vi "CC Focus GUI.vi"(9 "Standalone":bool=TRUE, 10 "Init Data":variant, 11 "Name":string) -> ()   [LabVIEW 2024]
uses:
  typedefs/CC enum Operation Mode.ctl
  Focus cluster Settings.ctl
  Focus Hardware Types.ctl
  Focus cluster Motion Settings.ctl
  Focus Class/Focus Class.lvclass
  Subsystems/SS typedef cluster Instrument Command Queue Data.ctl
  Subsystems/SS cluster Data Queue type.ctl
  Focus cluster MoveFocus Command Parameters.ctl
  hk-channel-class/hk-channel-class/HK Item/HK Item.lvclass
  FocusSimulator/FocusSimulator.lvclass
  NewFocus/NewFocus.lvclass
  ArduinoFocus/ArduinoFocus.lvclass
  hk-channel-class/hk-channel-class/HK Item/HK Item.lvclass/HK Item.ctl
  hk-channel-class/hk-channel-class/HK Item/HK Channel cluster Telemetry Data.ctl
  hk-channel-class/hk-channel-class/HK Item/HK Channel enum Data Type.ctl
  typedefs/CC cluster Script.ctl
  typedefs/CC Script Step.ctl
  typedefs/CC enum Script Action.ctl
  Scripts/CC Rd Wr Script Action.ctl
  hk-channel-class/hk-channel-class/HK Item/Write Source.vi
  hk-channel-class/hk-channel-class/HK Item/HK Channel Read Name.vi
panel:
  out "Messages":string
  in  "Mode":T1
  in  "Tab Control":enum32{"Focus Motor", "Engineering"}(tab)
  in  "Exp Time":dbl format="%.1g"
  in  "Peform Focus Scan":bool
  in  "Images":i32=10
  in  "Motor 1 Steps":i32
  in  "Motor 0 Steps":i32
  in  "Absolute":bool
  in  "Relative":bool
  in  "Steps":i32
  out "Controller Name":string
  in  "Select Motor (0:n-1)":i32 min=0 max=3 step=1
  out "Positions":i32[](array[slide]) scale=-10000.0..10000.0
  in  "Error":bool
  out "Homed":bool[](array[boolean])
  in  "STOP":bool
  out "Connected":bool
  in  "Close":bool
  in  "Home":bool
  in  "Configure":bool
  in  "Reset Startup Positions":bool
  in  "Connect":bool
  in  "Focus Settings":T2
  in  "Power Up Positions":i32[](array[numeric])
  # "Click for info"
  # "We need to remember where we were last in case\npower cycled on NewFocus controller. Change\ncode to use saved positions only if controller reports\nall 0s for position."
  # "Factory Settings: \nVelocity 1750 Steps/sec\nAcceleration 100000 Steps/sec/sec"
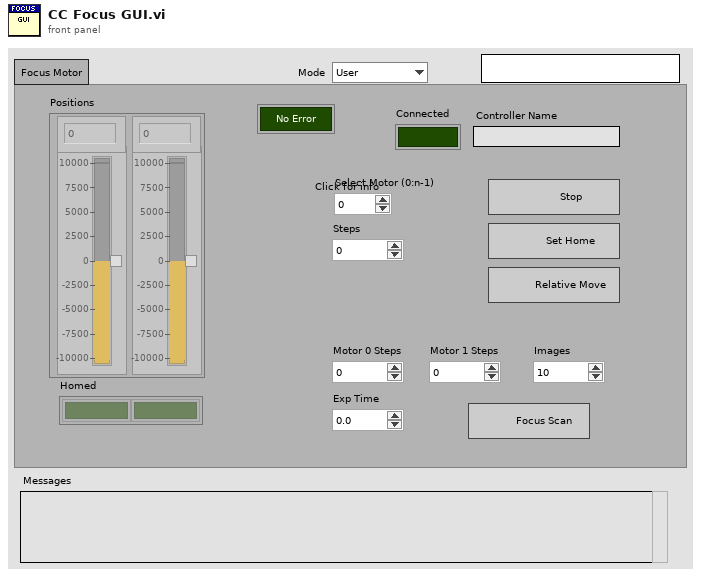
[diagram p1: front panel]
types:
  T1 = typedef "CC enum Operation Mode.ctl" = enum16{"User", "Engineering"}
  T2 = typedef "Focus cluster Settings.ctl" = cluster{"Type":T3, "Motion Settings":T4, "Last Positions":i32[]}
  T3 = typedef "Focus Hardware Types.ctl" = enum16{"Simulated", "NewFocus", "Arduino"}
  T4 = typedef "Focus cluster Motion Settings.ctl" = cluster{"Steps Per Sec":i32, "Steps Per Sec 2":i32}
  T5 = typedef "SS typedef cluster Instrument Command Queue Data.ctl" = cluster{"Cmd":string, "Parameters":variant}
  T6 = typedef "Focus cluster MoveFocus Command Parameters.ctl" = cluster{"Motor":i32, "Position":i32}
  T7 = cluster{"state":refnum<user-event>, "Focus Settings":T2, "Focus Ref":refnum<class "Focus Class.lvclass">, "Error":errorcluster, "Msg":string, "Start Pos":i32[], "cmd q":refnum<queue>, "data q":refnum<queue>, "next poll":timestamp, "Cmd":T5, "move":T6, "Name":string, "send time":timestamp, "Focus Script":string, "Ch List":refnum<class "HK Item.lvclass">[], "move names":string[], "pos names":string[], "Prev data":i32[]}
  T8 = typedef "SS cluster Data Queue type.ctl" = cluster{"Source":string, "Type":string, "Data":variant}
  T9 = typedef "HK Item.lvclass/HK Channel enum Data Type.ctl" = enum16{"Floating Point", "Integer", "Enum", "String", "Waveform", "File"}
  T10 = typedef "HK Item.lvclass/HK Channel cluster Telemetry Data.ctl" = cluster{"Ch Names":string[], "Ch Values":dbl[], "Timestamp":timestamp, "Data Type":T9}
  T11 = typedef "CC Rd Wr Script Action.ctl" = enum16{"Read", "Write", "List", "Delete"}
  T12 = typedef "CC cluster Script.ctl" = cluster{"Name":string, "Script":T13[]}
  T13 = typedef "CC Script Step.ctl" = cluster{"Action":T14, "Data":variant}
  T14 = typedef "CC enum Script Action.ctl" = enum16{"Noop", "Define Object", "Define Exposure", "Define Dithering", "Acquire Images", "Set Filter Wheel", "Telescope Home", "Telescope Move", "Telescope RA DEC", "Focus Move Relative", "Focus Move Absolute", "Focus Set Home", "Macro", "Pause", "Ask User", "Define Random Dither", "CmdLine", "Outlet"}
  T15 = typedef "CC cluster Script Panel Defaults.ctl" = cluster{"Script Name":string, "Script Path":path}
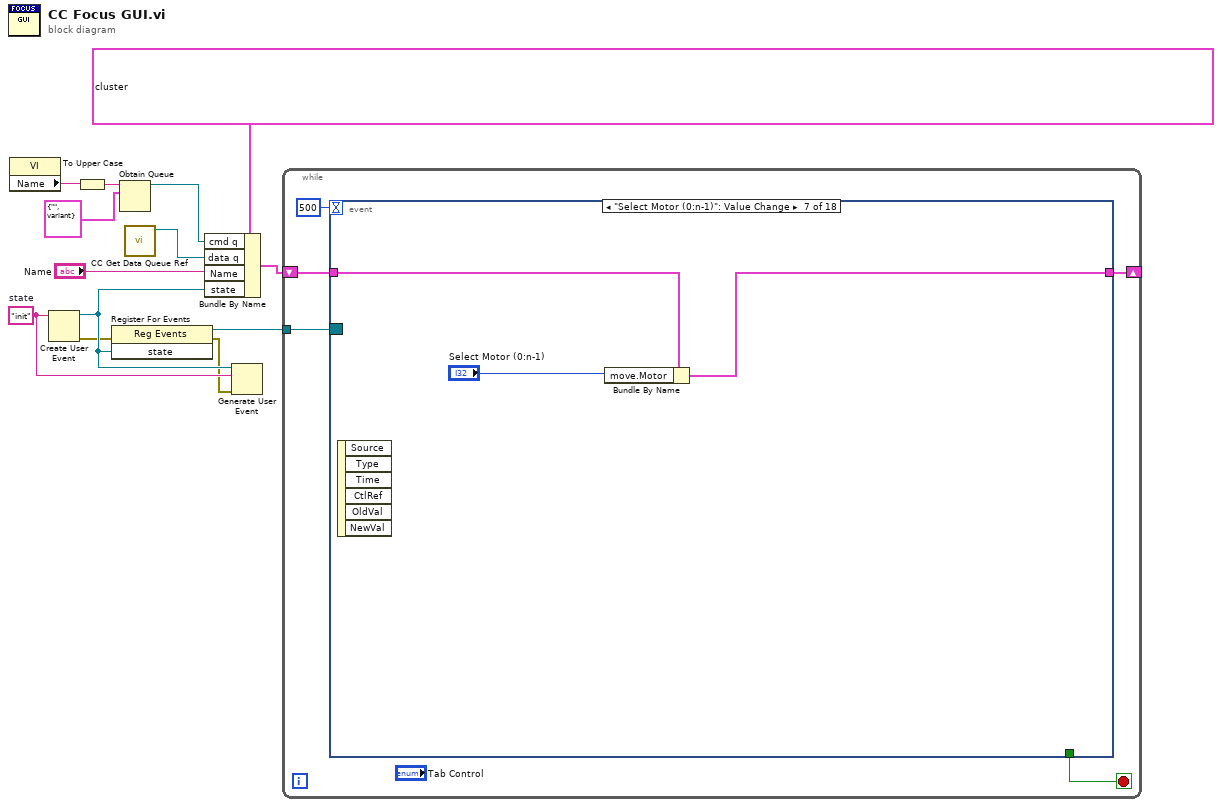
[diagram p0: block diagram]
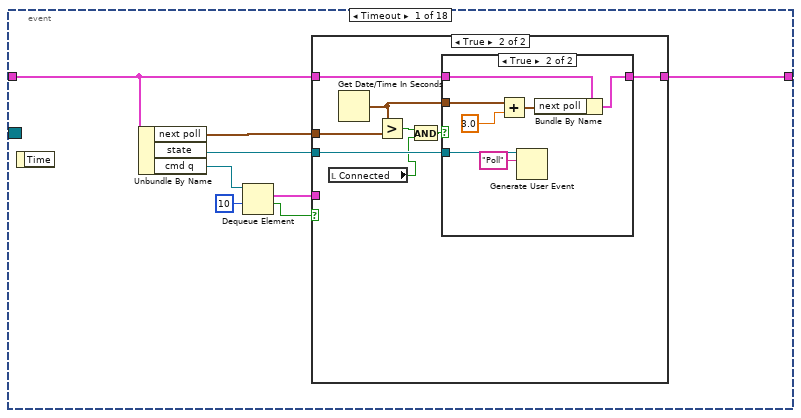
[diagram p2: hidden frame]
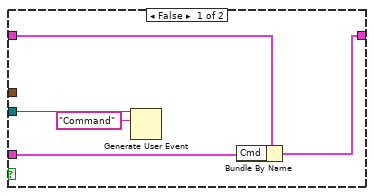
[diagram p3: hidden frame]
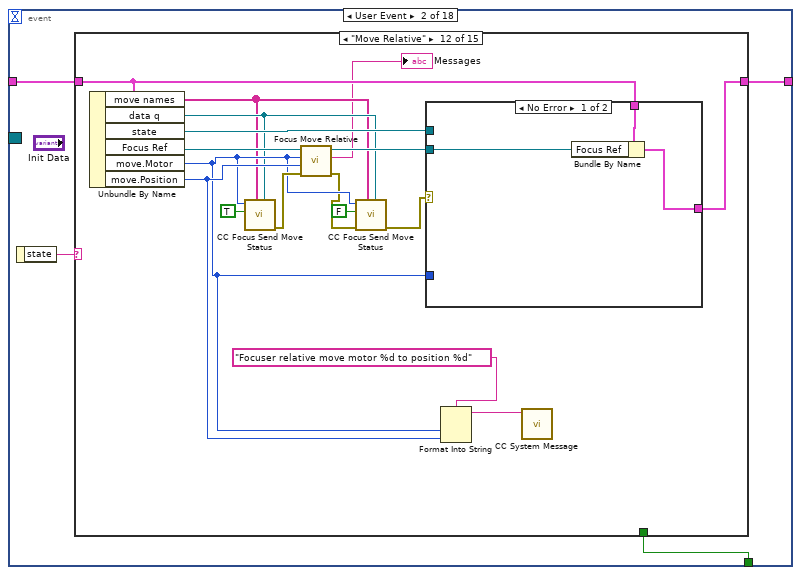
[diagram p5: hidden frame]
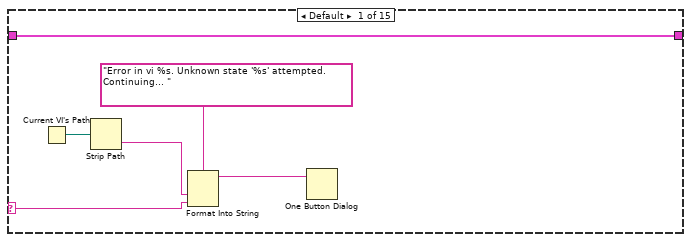
[diagram p6: hidden frame]
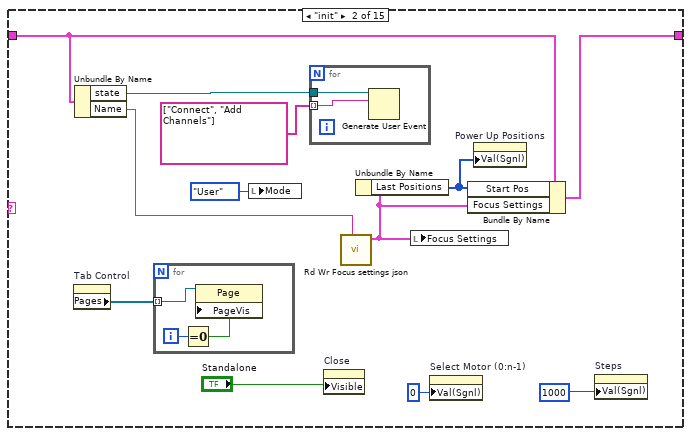
[diagram p7: hidden frame]
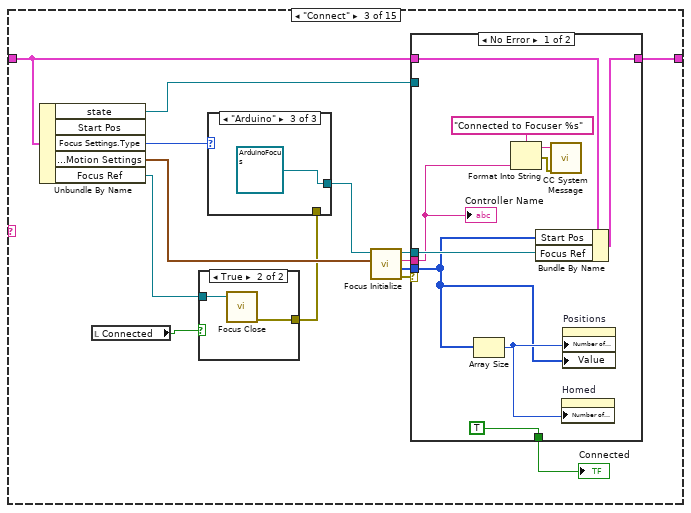
[diagram p8: hidden frame]
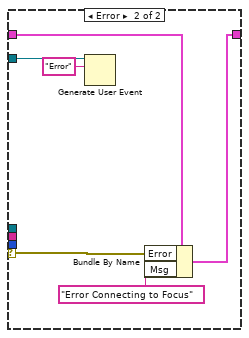
[diagram p10: hidden frame]
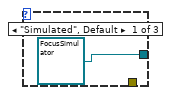
[diagram p11: hidden frame]
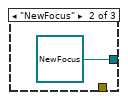
[diagram p12: hidden frame]
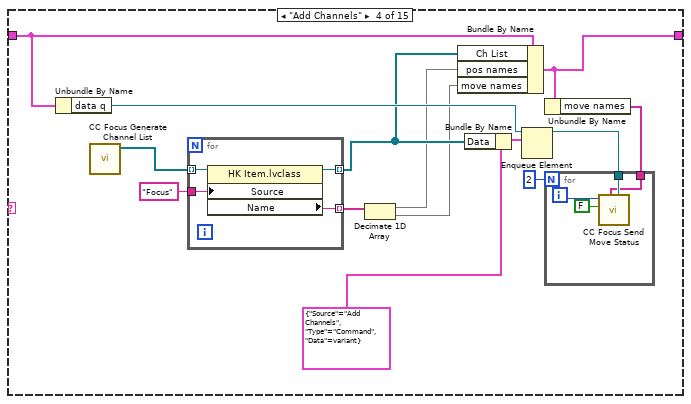
[diagram p13: hidden frame]
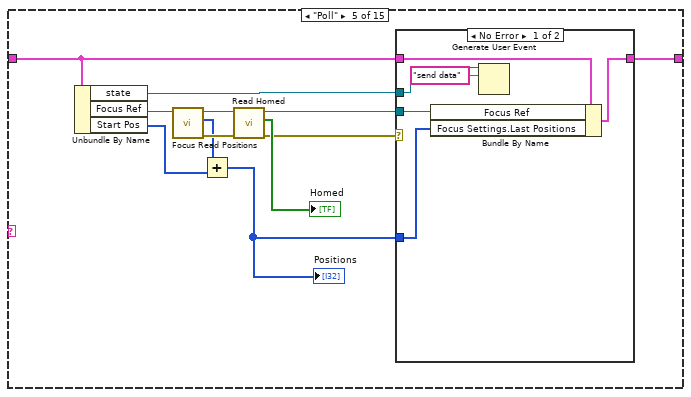
[diagram p14: hidden frame]
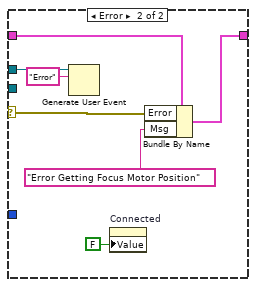
[diagram p15: hidden frame]
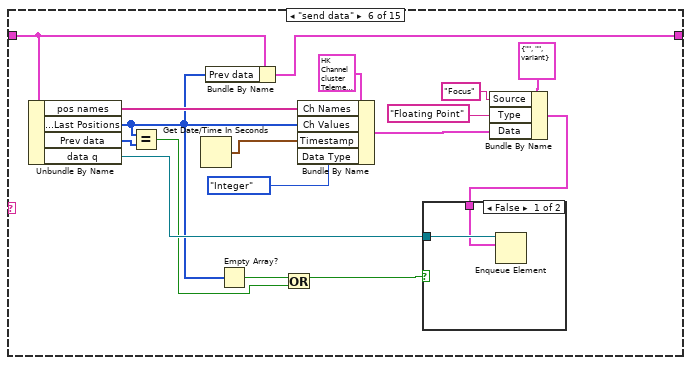
[diagram p16: hidden frame]
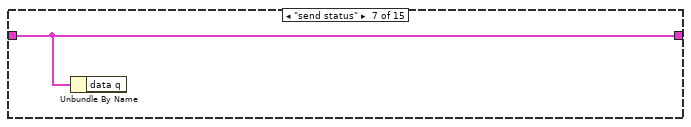
[diagram p18: hidden frame]
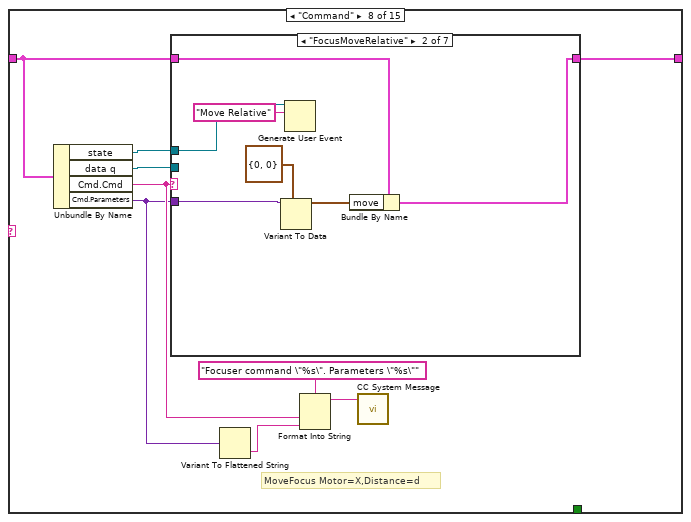
[diagram p19: hidden frame]
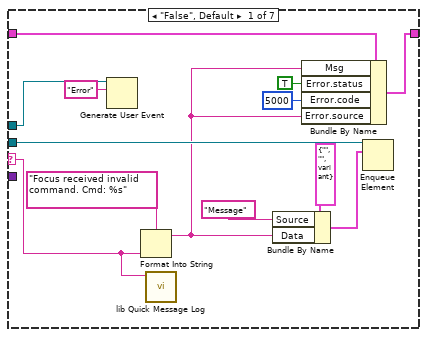
[diagram p20: hidden frame]
diagram:
  w9 = "init"  # state
  n1 = property class="VI"() -> ("Name"=w6:string)  [unwired: 2 in, 2 out]
  n2 = Create User Event(user event datatype=w9) -> (user event=w11:refnum<user-event>, error out=w7:errorcluster)  [unwired: 1 in]
  n3 = To Upper Case(1:w6) -> (0:w5:string)
  n4 = register-events(error in=w7, w11) -> (reference out=w10:refnum<event-registration>, error out=w8:errorcluster)  [unwired: 1 in]
  n5 = Obtain Queue(name (unnamed)=w5, element data type=T5 {"Cmd"="", "Parameters"=variant}) -> (queue out=w3:refnum<queue>)  [unwired: 3 in, 2 out]
  n6 = call "CC Get Data Queue Ref.vi"() -> ("Data Q"=w2:refnum<queue>)  [unwired: 10 in, 1 out]
  n7 = Bundle By Name(cluster=T7 {"state"=refnum, "Focus Settings"={"Type"=enum."Simulated", "Motion Settings"={"Steps Per Sec"=0, "Steps Per Sec 2"=0}, "Last Positions"=[]}, "Focus Ref"=refnum, "Error"={"status"=FALSE, "code"=0, "source"=""}, "Msg"="", "Start Pos"=[], "cmd q"=refnum, "data q"=refnum, "next poll"=timestamp(0 s since 1904-01-01), "Cmd"={"Cmd"="", "Parameters"=variant}, "move"={"Motor"=0, "Position"=0}, "Name"="NewFocus", "send time"=timestamp(0 s since 1904-01-01), "Focus Script"="", "Ch List"=[], "move names"=[], "pos names"=[], "Prev data"=[]}, "cmd q"=w3, "data q"=w2, "Name"="Name", "state"=w11) -> (w12:T7)
  n8 = Generate User Event(user event=w11, event data cluster=w9, error in=w8) -> ()  [unwired: 1 in, 2 out]
  n9 = while {
    tunnel: w10 -> [w18]
    shift-right: [w16] -> _
    shift-left: w12 -> [w17]
    stop <- w15 stop-if-true
    n10 = event shown="[6] \"Select Motor (0:n-1)\": Value Change" {
      selector: w18 -> [_ _ _ _ _ _ _ _ _ _ _ _ _ _ _ _ _ _]
      dyn-events: _ -> [_ _ _ _ _ _ _ _ _ _ _ _ _ _ _ _ _ _]
      timeout: 500 -> [_ _ _ _ _ _ _ _ _ _ _ _ _ _ _ _ _ _]
      tunnel: w17 -> [w20 w50 w338 w356 w362 w374 w378 w381 w387 w390 w393 w396 w397 w407 w417 w420 w434 w437]
      tunnel: [w19 w49 w340 w357 w362 w375 w379 w382 w387 w390 w393 w396 w398 w408 w417 w421 w434 w437] -> w16
      tunnel: [_ w48 _ _ _ _ _ _ _ _ _ _ _ _ _ _ _ _] -> w15
      event Timeout {
        n11 = event-data() -> ()  [unwired: 1 in, 1 out]
        n12 = Unbundle By Name(w20) -> ("next poll"=w21:timestamp, "state"=w22:refnum<user-event>, "cmd q"=w26:refnum<queue>)
        n13 = Dequeue Element(queue=w26, timeout in ms (-1)=10) -> (element=w23:T5, timed out?=w24:bool)  [unwired: 1 in, 2 out]
        n14 = case shown="True" w24 {
          tunnel: w23 -> [w28 _]
          tunnel: w22 -> [w31 w36]
          tunnel: w20 -> [w29 w37]
          tunnel: [w27 w34] -> w19
          tunnel: w21 -> [_ w39]
          frame False {
            n15 = Generate User Event(user event=w31, event data cluster="Command" ("event data")) -> ()  [unwired: 2 in, 2 out]
            n16 = Bundle By Name(cluster=w29, "Cmd"=w28) -> (w27:T7)
          }
          frame True {
            n17 = local read "Connected"() -> (w32:bool)
            n18 = Get Date/Time In Seconds() -> (seconds since 1Jan1904=w35:timestamp)
            n19 = Greater?(x=w35, y=w39) -> (0:w38:bool)
            n20 = And(x=w38, y=w32) -> (x .and. y?=w33:bool)
            n21 = case shown="True" w33 {
              tunnel: w37 -> [w40 w47]
              tunnel: w36 -> [_ w46]
              tunnel: w35 -> [_ w45]
              tunnel: [w40 w42] -> w34
              frame False {
              }
              frame True {
                n22 = Add(x=w45, y=3.0) -> (x+y=w43:timestamp)
                n23 = Generate User Event(user event=w46, event data cluster="Poll" ("event data")) -> ()  [unwired: 2 in, 2 out]
                n24 = Bundle By Name(cluster=w47, "next poll"=w43) -> (w42:T7)
              }
            }
          }
        }
      }
      event User Event {
        n25 = event-data() -> ("state"=w51:string)  [unwired: 1 in]
        n26 = case shown="\"Move Relative\"" w51 {
          selector: w51 -> [w56 _ _ _ _ _ _ _ _ _ _ _ _ _ _]
          tunnel: w50 -> [w52 w66 w84 w118 w137 w157 w176 w182 w234 w241 w259 w287 w307 w328 w335]
          tunnel: [w52 w67 w85 w112 w136 w158 w176 w183 w234 w242 w260 w288 w308 w328 w335] -> w49
          tunnel: [_ _ _ _ _ _ _ _ _ _ _ _ _ TRUE _] -> w48
          frame Default {
            n27 = Current VI's Path() -> (path=w55:path)
            n28 = Strip Path(path=w55) -> (name=w54:string)  [unwired: 1 out]
            n29 = Format Into String(format string="Error in vi %s. Unknown state '%s' attempted. Continuing... ", w54, w56) -> (resulting string=w53:string)  [unwired: 2 in, 1 out]
            n30 = One Button Dialog(message=w53) -> ()  [unwired: 1 in, 1 out]
          }
          frame "init" {
            n31 = property on="Tab Control" class="TabCtl (strict)"() -> ("Pages"=w58:refnum<vi>[])  [unwired: 2 in, 2 out]
            n32 = Unbundle By Name(w66) -> ("state"=w69:refnum<user-event>, "Name"=w60:string)
            n33 = for {
              tunnel: w58 -> [w72] mode=indexing
              i -> [w71]
              n34 = Equal To 0?(x=w71) -> (x = 0?=w70:bool)
              n35 = property class="Page"(reference=w72, "PageVis"=w70) -> ()  [unwired: 1 in, 2 out]
            }
            n36 = local write "Mode"(CC_enum_Operation_Mode."User" ("Mode")) -> ()
            n37 = for {
              tunnel: w69 -> [w74]
              tunnel: string[] ["Connect", "Add Channels"] -> [w73] mode=indexing
              n38 = Generate User Event(user event=w74, event data cluster=w73) -> ()  [unwired: 2 in, 2 out]
            }
            n39 = property on="Close" class="Bool"("Visible"="Standalone") -> ()  [unwired: 2 in, 2 out]
            n40 = call "Rd Wr Focus settings json.vi"("Focus Name"=w60) -> ("Focus Settings"=w62:T2)  [unwired: 9 in, 1 out]
            n41 = Unbundle By Name(w62) -> ("Last Positions"=w61:i32[])
            n42 = local write "Focus Settings"(w62) -> ()
            n43 = property on="Select Motor (0:n-1)" class="DigNum (strict)"("Val(Sgnl)"=0 ("Value (Signaling)")) -> ()  [unwired: 2 in, 2 out]
            n44 = Bundle By Name(cluster=w66, "Start Pos"=w61, "Focus Settings"=w62) -> (w67:T7)
            n45 = property on="Power Up Positions" class="Arr (strict)"("Val(Sgnl)"=w61) -> ()  [unwired: 2 in, 2 out]
            n46 = property on="Steps" class="DigNum (strict)"("Val(Sgnl)"=1000 ("Steps")) -> ()  [unwired: 2 in, 2 out]
          }
          frame "Connect" {
            n47 = Unbundle By Name(w84) -> ("state"=w81:refnum<user-event>, "Focus Settings.Type"=w88:T3, "Focus Settings.Motion Settings"=w83:T4, "Focus Ref"=w77:refnum<class "Focus Class.lvclass">)  [unwired: 1 out]
            n48 = local read "Connected"() -> (w78:bool)
            n49 = case shown="True" w78 {
              tunnel: w77 -> [_ w90]
              tunnel: [_ w89] -> w76
              frame False {
              }
              frame True {
                n50 = call-dynamic "Focus Close.vi"("Focus Class in"=w90) -> ("error out"=w89:errorcluster)  [unwired: 9 in, 1 out]
              }
            }
            n51 = case shown="\"Arduino\"" w88 {
              tunnel: [refnum<class "FocusSimulator.lvclass"> refnum ("FocusSimulator.lvclass") refnum<class "NewFocus.lvclass"> refnum ("NewFocus.lvclass") refnum<class "ArduinoFocus.lvclass"> refnum ("ArduinoFocus.lvclass")] -> w87
              tunnel: w76 -> [_ _ _]
              frame "Simulated", Default {
              }
              frame "NewFocus" {
              }
              frame "Arduino" {
              }
            }
            n52 = call-dynamic "Focus Initialize.vi"("Motion Settings"=w83, "Focus Class in"=w87) -> ("error out"=w82:errorcluster, "Motor Positions"=w75:i32[], "Device Name"=w80:string, "Focus Class out"=w86:refnum<class "Focus Class.lvclass">)  [unwired: 6 in]
            n53 = case shown="No Error" w82 {
              selector: w82 -> [_ w105]
              tunnel: w86 -> [w100 _]
              tunnel: [w99 w104] -> w85
              tunnel: w84 -> [w98 w106]
              tunnel: w81 -> [_ w103]
              tunnel: w80 -> [w93 _]
              tunnel: [TRUE _] -> w79
              tunnel: w75 -> [w91 _]
              frame No Error {
                n54 = Array Size(array=w91) -> (size(s)=w92:i32)
                n55 = Format Into String(format string="Connected to Focuser %s", w93) -> (resulting string=w94:string, error out=w96:errorcluster)  [unwired: 2 in]
                n56 = Bundle By Name(cluster=w98, "Start Pos"=w91, "Focus Ref"=w100) -> (w99:T7)
                n57 = call "CC System Message.vi"("error in (no error)"=w96, "Message"=w94) -> ()  [unwired: 9 in, 1 out]
                n58 = property on="Homed" class="Arr (strict)"("Number of Columns"=w92) -> ()  [unwired: 2 in, 2 out]
                n59 = property on="Positions" class="Arr (strict)"("Number of Columns"=w92, "Value"=w91) -> ()  [unwired: 2 in, 2 out]
                "Controller Name" <- w93
              }
              frame Error {
                n60 = Generate User Event(user event=w103, event data cluster="Error" ("event data")) -> ()  [unwired: 2 in, 2 out]
                n61 = Bundle By Name(cluster=w106, "Error"=w105, "Msg"="Error Connecting to Focus") -> (w104:T7)
              }
            }
            "Connected" <- w79
          }
          frame "Add Channels" {
            n62 = Unbundle By Name(w118) -> ("data q"=w121:refnum<queue>)
            n63 = call "CC Focus Generate Channel List.vi"() -> ("Channel List"=w117:refnum<class "HK Item.lvclass">[])  [unwired: 9 in, 2 out]
            n64 = for {
              tunnel: w117 -> [w131] mode=indexing
              tunnel: [w130] -> w120 mode=indexing
              tunnel: "Focus" ("Name") -> [w129]
              tunnel: [w128] -> w116 mode=indexing
              n65 = property class="HK Item.lvclass"(reference=w131, "Source"=w129) -> (reference out=w130:refnum<class "HK Item.lvclass">, "Name"=w128:string)  [unwired: 1 in, 1 out]
            }
            n66 = Decimate 1D Array(w116) -> (w115:string[], w114:string[])
            n67 = Bundle By Name(cluster=w118, "Ch List"=w120, "pos names"=w115, "move names"=w114) -> (w112:T7)
            n68 = Bundle By Name(cluster=T8 {"Source"="Add Channels", "Type"="Command", "Data"=variant} ("element"), "Data"=w120) -> (w123:T8)
            n69 = Enqueue Element(queue=w121, element=w123) -> (queue out=w113:refnum<queue>)  [unwired: 2 in, 2 out]
            n70 = Unbundle By Name(w112) -> ("move names"=w111:string[])
            n71 = for {
              N: 2 -> [_]
              tunnel: w113 -> [w126]
              tunnel: w111 -> [w124]
              i -> [w125]
              n72 = call "CC Focus Send Move Status.vi"("data q"=w126, "Names"=w124, "Moving"=FALSE, "motor"=w125) -> ()  [unwired: 7 in, 1 out]
            }
          }
          frame "Poll" {
            n73 = Unbundle By Name(w137) -> ("state"=w138:refnum<user-event>, "Focus Ref"=w143:refnum<class "Focus Class.lvclass">, "Start Pos"=w132:i32[])
            n74 = call-dynamic "Focus Read Positions.vi"("Focus Class in"=w143) -> ("error out"=w141:errorcluster, "Motor Positions"=w134:i32[], "Focus Class out"=w142:refnum<class "Focus Class.lvclass">)  [unwired: 8 in]
            n75 = Add(x=w134, y=w132) -> (x+y=w133:i32[])
            "Positions" <- w133
            n76 = call-dynamic "Read Homed.vi"("error in (no error)"=w141, "Focus Class in"=w142) -> ("error out"=w139:errorcluster, "Homed"=→"Homed":bool[], "Focus Class out"=w135:refnum<class "Focus Class.lvclass">)  [unwired: 7 in]
            n77 = case shown="No Error" w139 {
              selector: w139 -> [_ w153]
              tunnel: w138 -> [w145 w155]
              tunnel: w137 -> [w147 w156]
              tunnel: [w148 w151] -> w136
              tunnel: w135 -> [w149 _]
              tunnel: w133 -> [w146 _]
              frame No Error {
                n78 = Bundle By Name(cluster=w147, "Focus Ref"=w149, "Focus Settings.Last Positions"=w146) -> (w148:T7)
                n79 = Generate User Event(user event=w145, event data cluster="send data" ("event data")) -> ()  [unwired: 2 in, 2 out]
              }
              frame Error {
                n80 = Generate User Event(user event=w155, event data cluster="Error" ("event data")) -> ()  [unwired: 2 in, 2 out]
                n81 = property on="Connected" class="Bool (strict)"("Value"=FALSE ("Connected")) -> ()  [unwired: 2 in, 2 out]
                n82 = Bundle By Name(cluster=w156, "Error"=w153, "Msg"="Error Getting Focus Motor Position") -> (w151:T7)
              }
            }
          }
          frame "send data" {
            n83 = Unbundle By Name(w157) -> ("pos names"=w163:string[], "Focus Settings.Last Positions"=w159:i32[], "Prev data"=w162:i32[], "data q"=w170:refnum<queue>)
            n84 = Equal?(x=w159, y=w162) -> (x = y?=w160:bool)
            n85 = Get Date/Time In Seconds() -> (seconds since 1Jan1904=w172:timestamp)
            n86 = Bundle By Name(cluster=w157, "Prev data"=w159) -> (w158:T7)
            n87 = Empty Array?(array=w159) -> (empty?=w164:bool)
            n88 = Or(x=w164, y=w160) -> (x .or. y?=w161:bool)
            n89 = Bundle By Name(cluster=T10 {"Ch Names"=[], "Ch Values"=[], "Timestamp"=timestamp(0 s since 1904-01-01), "Data Type"=enum."Floating Point"}, "Ch Names"=w163, "Ch Values"=w159, "Timestamp"=w172, "Data Type"=HK_Channel_enum_Data_Type."Integer") -> (w166:T10)
            n90 = Bundle By Name(cluster=T8 {"Source"="", "Type"="", "Data"=variant} ("element"), "Source"="Focus", "Type"="Floating Point" ("Data Type"), "Data"=w166) -> (w165:T8)
            n91 = case shown="False" w161 {
              tunnel: w170 -> [w175 _]
              tunnel: w165 -> [w174 _]
              frame False {
                n92 = Enqueue Element(queue=w175, element=w174) -> ()  [unwired: 2 in, 3 out]
              }
              frame True {
              }
            }
          }
          frame "send status" {
            n93 = Unbundle By Name(w176) -> ()  [unwired: 1 out]
          }
          frame "Command" {
            # "MoveFocus Motor=X,Distance=d"
            n94 = Unbundle By Name(w182) -> ("state"=w184:refnum<user-event>, "data q"=w185:refnum<queue>, "Cmd.Cmd"=w179:string, "Cmd.Parameters"=w178:variant)
            n95 = case shown="\"FocusMoveRelative\"" w179 {
              selector: w179 -> [w193 _ _ _ _ _ _]
              tunnel: w185 -> [w198 _ _ _ _ _ _]
              tunnel: w178 -> [_ w205 w212 w219 _ _ _]
              tunnel: w184 -> [w189 w201 w208 w216 w222 w224 w228]
              tunnel: w182 -> [w192 w203 w210 w218 w220 w223 w226]
              tunnel: [w187 w202 w209 w217 w220 w223 w226] -> w183
              frame "False", Default {
                n96 = Generate User Event(user event=w189, event data cluster="Error" ("event data")) -> ()  [unwired: 2 in, 2 out]
                n97 = Format Into String(format string="Focus received invalid command. Cmd: %s", w193) -> (resulting string=w186:string)  [unwired: 2 in, 1 out]
                n98 = call "lib Quick Message Log.vi"("Message"=w193) -> ()  [unwired: 9 in, 2 out]
                n99 = Bundle By Name(cluster=T8 {"Source"="", "Type"="", "Data"=variant} ("element"), "Source"="Message" ("Data Type"), "Data"=w186) -> (w194:T8)
                n100 = Bundle By Name(cluster=w192, "Msg"=w186, "Error.status"=TRUE ("error.status"), "Error.code"=5000 ("error.code"), "Error.source"=w186) -> (w187:T7)
                n101 = Enqueue Element(queue=w198, element=w194) -> ()  [unwired: 2 in, 3 out]
              }
              frame "FocusMoveRelative" {
                n102 = Variant To Data(type=T6 {"Motor"=0, "Position"=0}, Variant=w205) -> (data=w199:T6)  [unwired: 1 in, 1 out]
                n103 = Generate User Event(user event=w201, event data cluster="Move Relative" ("event data")) -> ()  [unwired: 2 in, 2 out]
                n104 = Bundle By Name(cluster=w203, "move"=w199) -> (w202:T7)
              }
              frame "FocusMoveAbsolute" {
                n105 = Variant To Data(type=T6 {"Motor"=0, "Position"=0}, Variant=w212) -> (data=w206:T6)  [unwired: 1 in, 1 out]
                n106 = Generate User Event(user event=w208, event data cluster="Move Absolute" ("event data")) -> ()  [unwired: 2 in, 2 out]
                n107 = Bundle By Name(cluster=w210, "move"=w206) -> (w209:T7)
              }
              frame "FocusSetHome" {
                n108 = Variant To Data(type=0 ("move.Motor"), Variant=w219) -> (data=w214:i32)  [unwired: 1 in, 1 out]
                n109 = Generate User Event(user event=w216, event data cluster="Set Home" ("event data")) -> ()  [unwired: 2 in, 2 out]
                n110 = Bundle By Name(cluster=w218, "move.Motor"=w214) -> (w217:T7)
              }
              frame "Status" {
                n111 = Generate User Event(user event=w222, event data cluster="Send Status" ("event data")) -> ()  [unwired: 2 in, 2 out]
              }
              frame "Config" {
                n112 = Generate User Event(user event=w224, event data cluster="Send Config" ("event data")) -> ()  [unwired: 2 in, 2 out]
              }
              frame "Shutdown" {
                n113 = Generate User Event(user event=w228, event data cluster="Shutdown" ("event data")) -> ()  [unwired: 2 in, 2 out]
              }
            }
            n114 = Variant To Flattened String(Variant=w178) -> (data string=w177:string)  [unwired: 1 out]
            n115 = Format Into String(format string="Focuser command \"%s\". Parameters \"%s\"", w179, w177) -> (resulting string=w180:string)  [unwired: 2 in, 1 out]
            n116 = call "CC System Message.vi"("Message"=w180) -> ()  [unwired: 10 in, 1 out]
          }
          frame "run focus scan" {
            n117 = Unbundle By Name(w234) -> ("Focus Script"=w233:string)
            n118 = call "CC Create Script Q.vi"() -> ("error out"=w230:errorcluster, "Script Q"=w232:refnum<queue>)  [unwired: 10 in]
            n119 = Bundle By Name(cluster=T5 {"Cmd"="", "Parameters"=variant} ("element"), "Cmd"="set script", "Parameters"=w233) -> (w238:T5)
            n120 = Enqueue Element(queue=w232, element=w238, error in (no error)=w230) -> (queue out=w237:refnum<queue>, error out=w235:errorcluster)  [unwired: 1 in, 1 out]
            n121 = Enqueue Element(queue=w237, element=T5 {"Cmd"="start script", "Parameters"=variant}, error in (no error)=w235) -> (queue out=w231:refnum<queue>, error out=w229:errorcluster)  [unwired: 1 in, 1 out]
            n122 = Release Queue(queue=w231, error in (no error)=w229) -> ()  [unwired: 1 in, 3 out]
          }
          frame "Stop" {
            n123 = Unbundle By Name(w241) -> ("Focus Ref"=w247:refnum<class "Focus Class.lvclass">, "move.Motor"=w245:i32)
            n124 = call-dynamic "Focus Stop.vi"("Motor (0:n-1)"=w245, "Focus Class in"=w247) -> ("Focus Class out"=w243:refnum<class "Focus Class.lvclass">)  [unwired: 8 in, 1 out]
            n125 = Bundle By Name(cluster=w241, "Focus Ref"=w243) -> (w242:T7)
            n126 = Format Into String(format string="Focuser stop motor %d" ("Message"), w245) -> (resulting string=w244:string)  [unwired: 2 in, 1 out]
            n127 = call "CC System Message.vi"("Message"=w244) -> ()  [unwired: 10 in, 1 out]
          }
          frame "Set Home" {
            n128 = Unbundle By Name(w259) -> ("state"=w261:refnum<user-event>, "Focus Ref"=w262:refnum<class "Focus Class.lvclass">, "move.Motor"=w251:i32, "data q"=w250:refnum<queue>, "move names"=w249:string[])
            n129 = call "CC Focus Send Move Status.vi"("data q"=w250, "Names"=w249, "Moving"=TRUE, "motor"=w251) -> ("error out"=w253:errorcluster)  [unwired: 7 in]
            n130 = call-dynamic "Focus Set Home.vi"("error in (no error)"=w253, "Motor (0:n-1)"=w251, "Focus Class in"=w262) -> ("error out"=w252:errorcluster, "Focus Class out"=w258:refnum<class "Focus Class.lvclass">)  [unwired: 7 in]
            n131 = call "CC Focus Send Move Status.vi"("data q"=w250, "Names"=w249, "error in (no error)"=w252, "Moving"=FALSE, "motor"=w251) -> ("error out"=w248:errorcluster)  [unwired: 6 in]
            n132 = Format Into String(format string="Focuser home motor %d" ("Message"), w251) -> (resulting string=w256:string)  [unwired: 2 in, 1 out]
            n133 = case shown="Error .." w248 {
              selector: w248 -> [_ w270]
              tunnel: w261 -> [_ w273]
              tunnel: w259 -> [w265 w271]
              tunnel: [w264 w269] -> w260
              tunnel: w251 -> [_ w267]
              tunnel: w258 -> [w263 _]
              frame No Error {
                n134 = Bundle By Name(cluster=w265, "Focus Ref"=w263) -> (w264:T7)
              }
              frame Error {
                n135 = Generate User Event(user event=w273, event data cluster="Error" ("event data")) -> ()  [unwired: 2 in, 2 out]
                n136 = Format Into String(format string="Error Setting Home Position on Focus Motor %d" ("Msg"), w267) -> (resulting string=w266:string)  [unwired: 2 in, 1 out]
                n137 = Bundle By Name(cluster=w271, "Error"=w270, "Msg"=w266) -> (w269:T7)
              }
            }
            n138 = call "CC System Message.vi"("Message"=w256) -> ()  [unwired: 10 in, 1 out]
          }
          frame "Move Relative" {
            n139 = Unbundle By Name(w287) -> ("move names"=w276:string[], "data q"=w277:refnum<queue>, "state"=w289:refnum<user-event>, "Focus Ref"=w290:refnum<class "Focus Class.lvclass">, "move.Motor"=w280:i32, "move.Position"=w283:i32)
            n140 = call "CC Focus Send Move Status.vi"("data q"=w277, "Names"=w276, "Moving"=TRUE, "motor"=w280) -> ("error out"=w281:errorcluster)  [unwired: 7 in]
            n141 = call-dynamic "Focus Move Relative.vi"("error in (no error)"=w281, "Counts"=w283, "Motor (0:n-1)"=w280, "Focus Class in"=w290) -> ("error out"=w278:errorcluster, "response"=→"Messages":string, "Focus Class out"=w286:refnum<class "Focus Class.lvclass">)  [unwired: 5 in]
            n142 = call "CC Focus Send Move Status.vi"("data q"=w277, "Names"=w276, "error in (no error)"=w278, "Moving"=FALSE, "motor"=w280) -> ("error out"=w275:errorcluster)  [unwired: 6 in]
            n143 = case shown="No Error" w275 {
              selector: w275 -> [_ w298]
              tunnel: w289 -> [_ w301]
              tunnel: w287 -> [w293 w299]
              tunnel: [w292 w297] -> w288
              tunnel: w280 -> [_ w295]
              tunnel: w286 -> [w291 _]
              frame No Error {
                n144 = Bundle By Name(cluster=w293, "Focus Ref"=w291) -> (w292:T7)
              }
              frame Error {
                n145 = Generate User Event(user event=w301, event data cluster="Error" ("event data")) -> ()  [unwired: 2 in, 2 out]
                n146 = Format Into String(format string="Error Moving motor %d" ("Msg"), w295) -> (resulting string=w294:string)  [unwired: 2 in, 1 out]
                n147 = Bundle By Name(cluster=w299, "Error"=w298, "Msg"=w294) -> (w297:T7)
              }
            }
            n148 = Format Into String(format string="Focuser relative move motor %d to position %d" ("Message"), w280, w283) -> (resulting string=w284:string)  [unwired: 2 in, 1 out]
            n149 = call "CC System Message.vi"("Message"=w284) -> ()  [unwired: 10 in, 1 out]
          }
          frame "Move Absolute" {
            n150 = Unbundle By Name(w307) -> ("state"=w309:refnum<user-event>, "Focus Ref"=w311:refnum<class "Focus Class.lvclass">, "move.Motor"=w303:i32, "move.Position"=w302:i32)
            n151 = call-dynamic "Focus Move Absolute.vi"("Position"=w302, "Motor (0:n-1)"=w303, "Focus Class in"=w311) -> ("error out"=w310:errorcluster, "Focus Class out"=w306:refnum<class "Focus Class.lvclass">)  [unwired: 7 in]
            n152 = case shown="No Error" w310 {
              selector: w310 -> [_ w319]
              tunnel: w309 -> [_ w322]
              tunnel: w307 -> [w314 w320]
              tunnel: [w312 w318] -> w308
              tunnel: w303 -> [_ w316]
              tunnel: w306 -> [w313 _]
              frame No Error {
                n153 = Bundle By Name(cluster=w314, "Focus Ref"=w313) -> (w312:T7)
              }
              frame Error {
                n154 = Generate User Event(user event=w322, event data cluster="Error" ("event data")) -> ()  [unwired: 2 in, 2 out]
                n155 = Format Into String(format string="Error Moving motor %d" ("Msg"), w316) -> (resulting string=w315:string)  [unwired: 2 in, 1 out]
                n156 = Bundle By Name(cluster=w320, "Error"=w319, "Msg"=w315) -> (w318:T7)
              }
            }
            n157 = Format Into String(format string="Focuser absoluite move motor %d to position %d" ("Message"), w303, w302) -> (resulting string=w304:string)  [unwired: 2 in, 1 out]
            n158 = call "CC System Message.vi"("Message"=w304) -> ()  [unwired: 10 in, 1 out]
          }
          frame "Shutdown" {
            n159 = Unbundle By Name(w328) -> ("Focus Settings"=w325:T2, "Focus Ref"=w327:refnum<class "Focus Class.lvclass">)
            n160 = call-dynamic "Focus Close.vi"("Focus Class in"=w327) -> ()  [unwired: 9 in, 2 out]
            n161 = call "Rd Wr Focus settings json.vi"("Write? (F:Read)"=TRUE, "Focus Settings"=w325) -> ()  [unwired: 8 in, 2 out]
            n162 = call "CC System Message.vi"("Message"="Focuser shutdown.") -> ()  [unwired: 10 in, 1 out]
          }
          frame "Error" {
            n163 = Unbundle By Name(w335) -> ("Error.status"=w334:bool, "Error.source"=w329:string, "Name"=w330:string)
            n164 = local write "Error"(w334) -> ()
            n165 = Format Into String(format string="Error connecting to focus motors %s. Error message: %s", w330, w329) -> (resulting string=w331:string, error out=w333:errorcluster)  [unwired: 2 in]
            n166 = call "CC System Message.vi"("error in (no error)"=w333, "Message"=w331) -> ()  [unwired: 9 in, 1 out]
          }
        }
      }
      event "Peform Focus Scan": Value Change {
        n167 = event-data() -> ()  [unwired: 1 in, 1 out]
        n168 = Unbundle By Name(w338) -> ("state"=w337:refnum<user-event>)
        n169 = Generate User Event(user event=w337, event data cluster="run focus scan" ("event data")) -> ()  [unwired: 2 in, 2 out]
        n170 = call "CC Focus Generate Focus Scan Script.vi"("Images"="Images", "Exp Time"="Exp Time", "Motor 0 Steps"="Motor 0 Steps", "Motor 1 Steps"="Motor 1 Steps") -> ("Script"=w341:T13[])  [unwired: 6 in, 1 out]
        n171 = Format Date/Time String(time format string (%c)="%Y%m%d_%H%M%S") -> (date/time string=w342:string)  [unwired: 2 in]
        n172 = Format Into String(format string="FocusScan_%s", w342) -> (resulting string=w339:string)  [unwired: 2 in, 1 out]
        n173 = Bundle By Name(cluster=T12 {"Name"="", "Script"=[]} ("Script"), "Name"=w339, "Script"=w341) -> (w350:T12)
        n174 = call "Rd Wr Script Defaults.vi"() -> ("Script Settings"=w349:T15)  [unwired: 10 in, 1 out]
        n175 = Unbundle By Name(w349) -> ("Script Path"=w348:path)
        n176 = Format Into String(format string="Created script %s.", w339) -> (resulting string=w344:string)  [unwired: 2 in, 1 out]
        n177 = call "CC Rd Wr Script.vi"("Script Path"=w348, "Action"=CC_Rd_Wr_Script_Action."Write", "Script"=w350) -> ()  [unwired: 3 in, 6 out]
        n178 = Bundle By Name(cluster=w338, "Focus Script"=w339) -> (w340:T7)
        n179 = call "CC System Message.vi"("Message"=w344) -> ()  [unwired: 10 in, 1 out]
      }
      event "Configure": Value Change {
        n180 = event-data() -> ()  [unwired: 1 in, 6 out]
        n181 = Unbundle By Name(w356) -> ("Focus Ref"=w359:refnum<class "Focus Class.lvclass">)
        n182 = call-dynamic "Focus Configure.vi"("Focus Class in"=w359) -> ("Focus Class out"=w358:refnum<class "Focus Class.lvclass">)  [unwired: 9 in, 1 out]
        n183 = Bundle By Name(cluster=w356, "Focus Ref"=w358) -> (w357:T7)
      }
      event Value Change {
        n184 = event-data() -> ()  [unwired: 1 in, 6 out]
        n185 = property on="Tab Control" class="TabCtl (strict)"() -> ("Pages"=w360:refnum<vi>[])  [unwired: 2 in, 2 out]
        n186 = case shown="\"User\", Default" "Mode" {
          tunnel: w360 -> [w363 w367]
          frame "User", Default {
            n187 = for {
              tunnel: w363 -> [w366] mode=indexing
              i -> [w365]
              n188 = Equal To 0?(x=w365) -> (x = 0?=w364:bool)
              n189 = property class="Page"(reference=w366, "PageVis"=w364) -> ()  [unwired: 1 in, 2 out]
            }
          }
          frame "Engineering" {
            n190 = for {
              tunnel: w367 -> [w369] mode=indexing
              n191 = property class="Page"(reference=w369, "PageVis"=TRUE ("Page Visible")) -> ()  [unwired: 1 in, 2 out]
            }
          }
        }
      }
      event Value Change {
        n192 = event-data() -> ()  [unwired: 1 in, 6 out]
        n193 = Unbundle By Name(w374) -> ("state"=w373:refnum<user-event>)
        n194 = for {
          tunnel: w373 -> [w377]
          tunnel: string[] ["Connect"] -> [w376] mode=indexing
          n195 = Generate User Event(user event=w377, event data cluster=w376) -> ()  [unwired: 2 in, 2 out]
        }
        n196 = call "Rd Wr Focus settings json.vi"("Write? (F:Read)"=TRUE, "Focus Settings"="Focus Settings") -> ()  [unwired: 8 in, 2 out]
        n197 = Bundle By Name(cluster=w374, "Focus Settings"="Focus Settings") -> (w375:T7)
      }
      event "Select Motor (0:n-1)": Value Change {
        n198 = event-data() -> ()  [unwired: 1 in, 6 out]
        n199 = Bundle By Name(cluster=w378, "move.Motor"="Select Motor (0:n-1)") -> (w379:T7)
      }
      event "Steps": Value Change {
        n200 = event-data() -> ("NewVal"=w383:i32)  [unwired: 1 in]
        n201 = Bundle By Name(cluster=w381, "move.Position"=w383) -> (w382:T7)
      }
      event "Connect": Value Change {
        n202 = event-data() -> ()  [unwired: 1 in, 6 out]
        n203 = Unbundle By Name(w387) -> ("state"=w385:refnum<user-event>, "Focus Ref"=w386:refnum<class "Focus Class.lvclass">)
        n204 = call-dynamic "Focus Close.vi"("Focus Class in"=w386) -> ()  [unwired: 9 in, 2 out]
        n205 = Generate User Event(user event=w385, event data cluster="Connect" ("event data")) -> ()  [unwired: 2 in, 2 out]
      }
      event "Home": Value Change {
        n206 = event-data() -> ()  [unwired: 1 in, 6 out]
        n207 = Unbundle By Name(w390) -> ("state"=w389:refnum<user-event>)
        n208 = Generate User Event(user event=w389, event data cluster="Set Home" ("event data")) -> ()  [unwired: 2 in, 2 out]
      }
      event "Relative": Value Change {
        n209 = event-data() -> ()  [unwired: 1 in, 6 out]
        n210 = Unbundle By Name(w393) -> ("state"=w392:refnum<user-event>)
        n211 = Generate User Event(user event=w392, event data cluster="Move Relative" ("event data")) -> ()  [unwired: 2 in, 2 out]
      }
      event "Absolute": Value Change {
        n212 = event-data() -> ()  [unwired: 1 in, 6 out]
        n213 = Unbundle By Name(w396) -> ("state"=w395:refnum<user-event>)
        n214 = Generate User Event(user event=w395, event data cluster="Move Absolute" ("event data")) -> ()  [unwired: 2 in, 2 out]
      }
      event "Power Up Positions": Value Change {
        n215 = event-data() -> ("NewVal"=w402:i32[])  [unwired: 1 in]
        n216 = Array Size(array=w402) -> (size(s)=w401:i32)
        n217 = Equal?(x=w401, y=3) -> (x = y?=w399:bool)
        n218 = case shown="False" w399 {
          tunnel: w397 -> [w405 w406]
          tunnel: [w403 w406] -> w398
          frame False {
            n219 = Bundle By Name(cluster=w405, "Start Pos"=i32[] [0, 0, 0] ("NewVal")) -> (w403:T7)
          }
          frame True {
          }
        }
      }
      event "Reset Startup Positions": Value Change {
        n220 = event-data() -> ()  [unwired: 1 in, 6 out]
        n221 = Array Size(array="Power Up Positions") -> (size(s)=w414:i32)
        n222 = Equal?(x=w414, y=3) -> (x = y?=w412:bool)
        n223 = Select(t="Power Up Positions", s=w412, f=i32[] [0, 0, 0] ("NewVal")) -> (s? t:f=w409:i32[])
        n224 = Bundle By Name(cluster=w407, "Start Pos"=w409) -> (w408:T7)
      }
      event "STOP": Value Change {
        n225 = event-data() -> ()  [unwired: 1 in, 6 out]
        n226 = Unbundle By Name(w417) -> ("state"=w416:refnum<user-event>)
        n227 = Generate User Event(user event=w416, event data cluster="Stop" ("event data")) -> ()  [unwired: 2 in, 2 out]
      }
      event "Error": Value Change {
        n228 = event-data() -> ("CtlRef"=w419:refnum<vi>)  [unwired: 1 in]
        n229 = Unbundle By Name(w420) -> ("Msg"=w422:string, "Error.code"=w427:i32, "Error.source"=w426:string, "Error.status"=w425:bool)
        n230 = Format Into String(format string="An error occurred during %s. \nError Number: %d\nError message: %s", w422, w427, w426) -> (resulting string=w424:string)  [unwired: 2 in, 1 out]
        n231 = call "Display Message to User"("Enable"=w425, "Message"=w424) -> ("error out"=w423:errorcluster, "Close"=w418:bool)  [unwired: 8 in]
        n232 = case shown="False" w418 {
          tunnel: w420 -> [w431 w432]
          tunnel: [w429 w432] -> w421
          tunnel: w423 -> [w430 _]
          frame False {
            n233 = Bundle By Name(cluster=w431, "Error"=w430) -> (w429:T7)
          }
          frame True {
          }
        }
        n234 = property class="Bool (strict)"(reference=w419, "Value"=w418) -> ()  [unwired: 1 in, 2 out]
      }
      event "Standalone": Value Change {
        n235 = event-data() -> ("NewVal"=w433:bool)  [unwired: 1 in]
        n236 = property on="Close" class="Bool"("Visible"=w433) -> ()  [unwired: 2 in, 2 out]
      }
      event "Close": Value Change {
        n237 = event-data() -> ()  [unwired: 1 in, 6 out]
        n238 = Unbundle By Name(w437) -> ("state"=w436:refnum<user-event>)
        n239 = Generate User Event(user event=w436, event data cluster="Shutdown" ("event data")) -> ()  [unwired: 2 in, 2 out]
      }
    }
  }
